vi "SDG60ConfArbWaveform2.vi"(5 "Select Channel (1:Channel 1)":i32(ring)=1 items=["Channel 1"=1, "Channel 2"=2], 6 "DC Offset (0.00 V)":dbl min=-10.0 max=10.0, 7 "Amplitude (1.0 Vpp)":dbl=1.0 min=0.001 max=20.0 step=1.0 format="%#.3f", 8 "error in (no error)":errorcluster, 9 "Phase (0.0 degrees)":dbl=0.002 min=-360.0 max=360.0 format="%#.1g", 10 "Frequency (1000 Hz)":dbl=1000.0 min=1e-06 max=160000000.0 step=1.0 format="%#.15g", 11 "VISA resource name":refnum<visa-resource-name>="USB0::0xF4EC::0x1101::SDG6XEBC5R0119::INSTR") -> ()   [LabVIEW 2018]
doc: "Sets the waveform parameters for an arbitrary waveform. This VI should be called after <b>Create Arbitrary Waveform.vi</b> (for user defined arbitrary waveform) and <b>Select Arbitrary Waveform.vi</b>"
panel:
  in  "Sample Rate (Sa/s)":dbl=1000.0 min=1.0 max=300000000.0 step=1.0 format="%#.15g"
  out "error out":errorcluster
  out "VISA resource name out":refnum<visa-resource-name>
  in  "DDS/TArb 0: DDS":u16(ring) items=["DDS", "TrueArb"]
  in  "Interpolation 0: Zero-order":u16(ring) items=["Zero-Order", "Linear"]
  # "Todo: sync"
  # "2mVpp-20Vpp"
  # "Will ignore selected interpolaton when using DDS\nMay take time to switch to TrueArb if WFM is large"
  # "Range: 1uHz-50MHz\n10 Digit precision"
  # "Range: 1uSa/s- 300 MSa/s\n10 Digit precision"
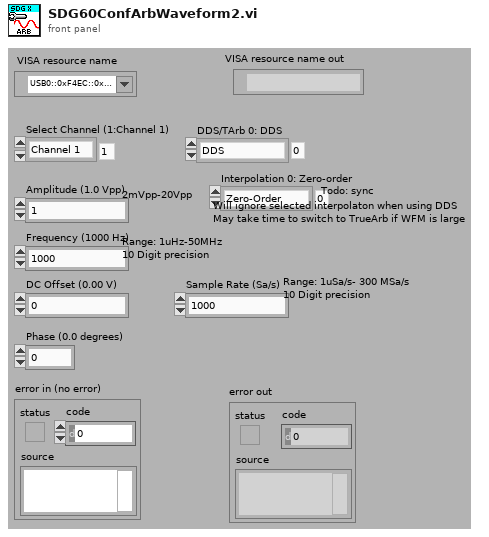
[diagram p1: front panel]
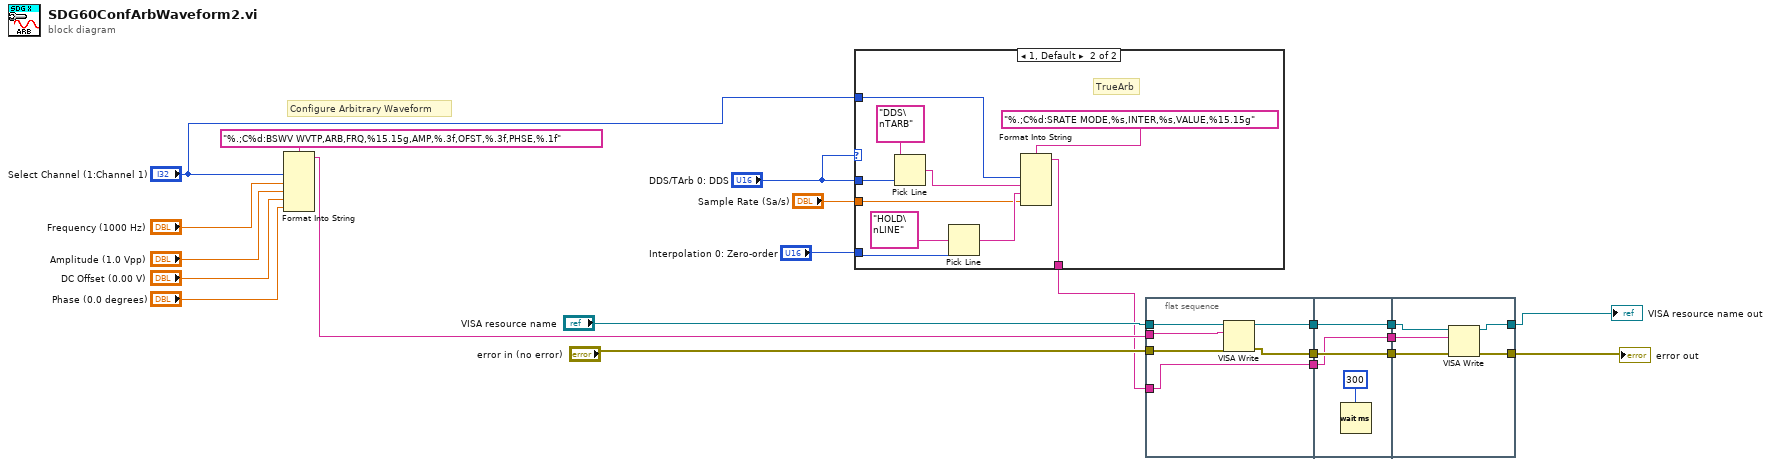
[diagram p0: block diagram]
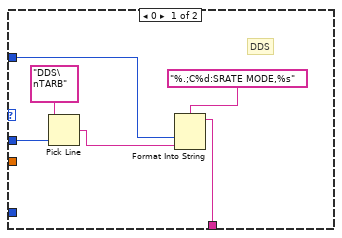
[diagram p2: hidden frame]
diagram:
  # "Configure Arbitrary Waveform"
  n1 = Format Into String(format string="%.;C%d:BSWV WVTP,ARB,FRQ,%15.15g,AMP,%.3f,OFST,%.3f,PHSE,%.1f", "Select Channel (1:Channel 1)", "Frequency (1000 Hz)", "Amplitude (1.0 Vpp)", "DC Offset (0.00 V)", "Phase (0.0 degrees)") -> (resulting string=w11:string)  [unwired: 2 in, 1 out]
  n2 = case shown="1, Default" "DDS/TArb 0: DDS" {
    tunnel: "Interpolation 0: Zero-order" -> [_ w36]
    tunnel: "DDS/TArb 0: DDS" -> [w26 w34]
    tunnel: "Select Channel (1:Channel 1)" -> [w24 w32]
    tunnel: [w23 w31] -> w5
    tunnel: "Sample Rate (Sa/s)" -> [_ w30]
    frame 0 {
      # "DDS"
      n3 = Pick Line(multi-line string="DDS\nTARB", line index=w26) -> (output string=w25:string)  [unwired: 1 in]
      n4 = Format Into String(format string="%.;C%d:SRATE MODE,%s", w24, w25) -> (resulting string=w23:string)  [unwired: 2 in, 1 out]
    }
    frame 1, Default {
      # "TrueArb"
      n5 = Pick Line(multi-line string="DDS\nTARB", line index=w34) -> (output string=w33:string)  [unwired: 1 in]
      n6 = Pick Line(multi-line string="HOLD\nLINE", line index=w36) -> (output string=w35:string)  [unwired: 1 in]
      n7 = Format Into String(format string="%.;C%d:SRATE MODE,%s,INTER,%s,VALUE,%15.15g", w32, w33, w35, w30) -> (resulting string=w31:string)  [unwired: 2 in, 1 out]
    }
  }
  n8 = flat-sequence {
    tunnel: [w41] -> w14
    tunnel: "VISA resource name" -> [w43]
    tunnel: w11 -> [w42]
    tunnel: "error in (no error)" -> [w40]
    tunnel: [w39] -> w7
    tunnel: w5 -> [w38]
    tunnel: [w38] -> w4
    tunnel: w14 -> [w46]
    tunnel: [w46] -> w13
    tunnel: [w45] -> w8
    tunnel: w7 -> [w45]
    tunnel: w4 -> [w44]
    tunnel: [w44] -> w3
    tunnel: [w48] -> w12
    tunnel: w13 -> [w49]
    tunnel: w8 -> [w52]
    tunnel: [w51] -> w6
    tunnel: w3 -> [w50]
    frame #0 {
      n9 = VISA Write(VISA resource name=w43, write buffer=w42, error in (no error)=w40) -> (VISA resource name out=w41:refnum<visa-resource-name>, error out=w39:errorcluster)  [unwired: 1 out]
    }
    frame #1 {
      n10 = Wait (ms)(milliseconds to wait=300 ("x")) -> ()  [unwired: 1 out]
    }
    frame #2 {
      n11 = VISA Write(VISA resource name=w49, write buffer=w50, error in (no error)=w52) -> (VISA resource name out=w48:refnum<visa-resource-name>, error out=w51:errorcluster)  [unwired: 1 out]
    }
  }
  "VISA resource name out" <- w12
  "error out" <- w6
